vi "Global 1.vi"() -> ()   [LabVIEW 2015]
panel:
  out "Reverse Mode":bool
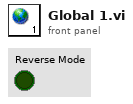
[diagram p1: front panel]
diagram:
